vi "rename channel test.vi"() -> ()   [LabVIEW 2013, in "Shared Library Module tests.lvlib"]
doc: "Platypus Framework 1.0.1.60\nNI Systems Engineering - National Instruments"
uses:
  Shared Library Module tests.lvlib
  <vilib>/NI/Tag Bus Module Framework/channel/channel classification.ctl
  configuration/Shared Library Module configuration.lvclass
  <vilib>/NI/Tag Bus/tag/tag descriptor.lvclass/tag descriptor.ctl
  <vilib>/NI/Tag Bus Module Framework/channel/TBM channel.lvclass
  <vilib>/NI/Tag Bus Module Framework/root configuration/TBM configuration.lvclass
  <vilib>/NI/Tag Bus/tag/tag descriptor.lvclass
panel:
  out "rename success":bool
  out "no err":errorcluster
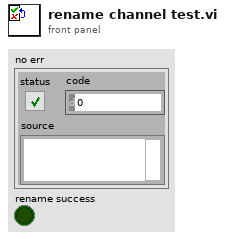
[diagram p1: front panel]
types:
  T1 = typedef "TBM channel.lvclass/channel classification.ctl" = enum16{"input data", "output data", "processing parameter", "processing result"}
  T2 = typedef "tag bus.lvlib/tag descriptor.lvclass/Data Type.ctl" = enum16{"Double", "Single", "I64", "I32", "I16", "I8", "U64", "U32", "U16", "U8", "Boolean", "String", "Array of Double", "Array of Single", "Array of I64", "Array of I32", "Array of I16", "Array of I8", "Array of U64", "Array of U32", "Array of U16", "Array of U8", "Array of Boolean", "Array of String"}
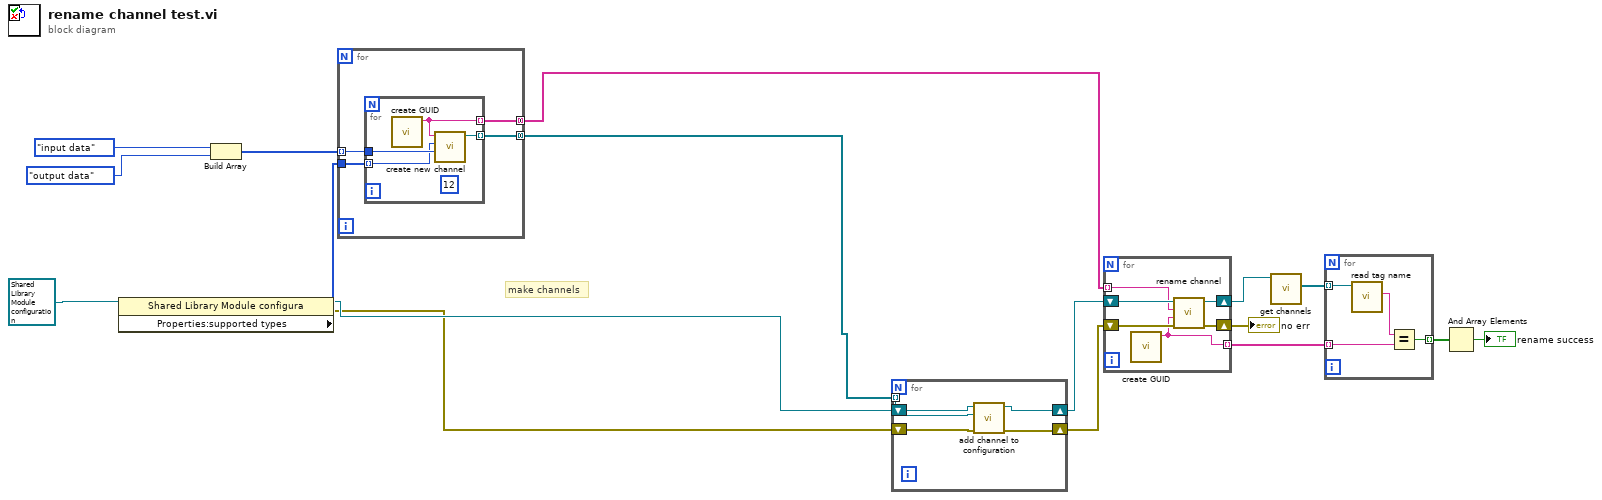
[diagram p0: block diagram]
diagram:
  # "make channels"
  n1 = property class="Shared Library Module configura"(reference=refnum<class "Shared Library Module configuration.lvclass"> refnum ("tag bus configurable plugin module configuration")) -> (reference out=w5:refnum<class "Shared Library Module configuration.lvclass">, error out=w1:errorcluster, "Properties:supported types"=w14:T2[])  [unwired: 1 in]
  n2 = Build Array(channel_classification."input data" ("channel classification"), channel_classification."output data" ("channel classification")) -> (w15:T1[])
  n3 = for {
    tunnel: w15 -> [w21] mode=indexing
    tunnel: [w19] -> w4 mode=concatenating
    tunnel: w14 -> [w20]
    tunnel: [w18] -> w13 mode=concatenating
    n4 = for {
      tunnel: w21 -> [w24]
      tunnel: [w25] -> w19 mode=indexing
      tunnel: w20 -> [w23] mode=indexing
      tunnel: [w22] -> w18 mode=indexing
      (unwired) 12
      n5 = call <vilib>:"create GUID.vi"() -> ("uuid"=w22:string)  [unwired: 11 in]
      n6 = call <vilib>:"create new channel.vi"("channel classification"=w24, "data type"=w23, "channel name"=w22) -> ("channel"=w25:refnum<class "TBM channel.lvclass">)  [unwired: 8 in]
    }
  }
  n7 = for {
    shift-right: [w29] -> w3
    shift-left: w5 -> [w30]
    shift-right: [w28] -> w2
    shift-left: w1 -> [w27]
    tunnel: w4 -> [w26] mode=indexing
    n8 = call "add channel to configuration.vi"("error in"=w27, "TBM channel in"=w26, "Shared Library Module configuration in"=w30) -> ("error out"=w28:errorcluster, "Shared Library Module configuration out"=w29:refnum<class "Shared Library Module configuration.lvclass">)  [unwired: 7 in]
  }
  n9 = for {
    tunnel: w13 -> [w32] mode=indexing
    shift-right: [w33] -> w12
    shift-left: w3 -> [w36]
    shift-right: [w34] -> w10
    shift-left: w2 -> [w35]
    tunnel: [w31] -> w11 mode=indexing
    n10 = call <vilib>:"create GUID.vi"() -> ("uuid"=w31:string)  [unwired: 11 in]
    n11 = call "rename channel.vi"("error in"=w35, "new name"=w31, "old name"=w32, "Shared Library Module configuration in"=w36) -> ("error out"=w34:errorcluster, "Shared Library Module configuration out"=w33:refnum<class "Shared Library Module configuration.lvclass">)  [unwired: 6 in]
  }
  "no err" <- w10
  n12 = call-dynamic "get channels.vi"("Shared Library Module configuration in"=w12) -> ("channels"=w9:refnum<class "TBM channel.lvclass">[])  [unwired: 9 in, 1 out]
  n13 = for {
    tunnel: w11 -> [w39] mode=indexing
    tunnel: w9 -> [w40] mode=indexing
    tunnel: [w37] -> w8 mode=indexing
    n14 = call <vilib>:"read tag name.vi"("system tag in"=w40) -> ("name"=w38:string)  [unwired: 8 in, 2 out]
    n15 = Equal?(x=w38, y=w39) -> (x = y?=w37:bool)
  }
  n16 = And Array Elements(Boolean array=w8) -> (logical AND=→"rename success":bool)
